vi "Nav_CheckMinDistanceToNode.vi"(9 "Array of path nodes":T1, 11 "Robot current position":T2) -> (3 "Coordinates":T1)   [LabVIEW 2009, in "Navigation.lvlib"]
uses:
  Navigation.lvlib
  Nav_CordinateArray.ctl
  Drive/Drive_Utils.lvlib
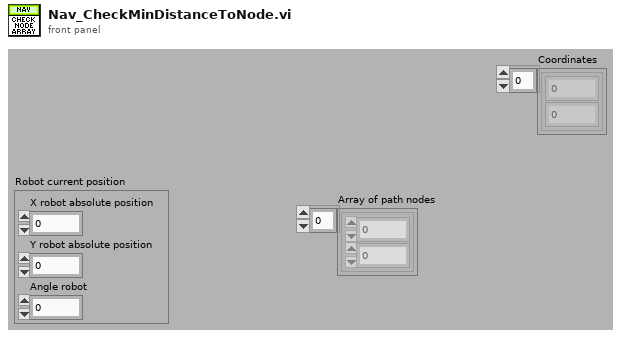
[diagram p1: front panel]
types:
  T1 = typedef "Navigation.lvlib/Nav_CordinateArray.ctl" = cluster{"X position":dbl, "Y position":dbl}[]
  T2 = cluster{"X robot absolute position":dbl, "Y robot absolute position":dbl, "Angle robot":dbl}
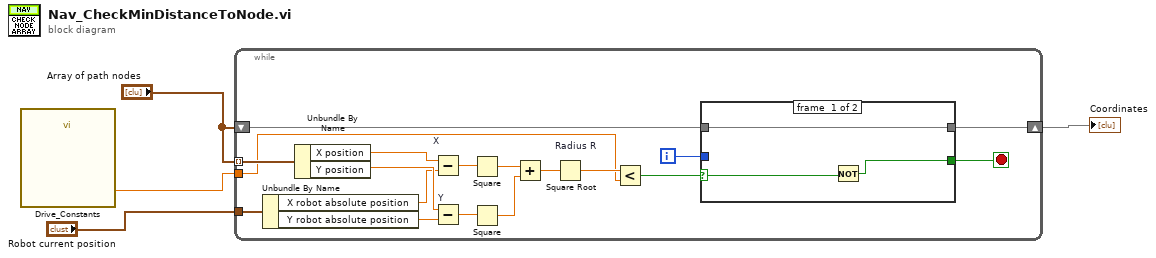
[diagram p0: block diagram]
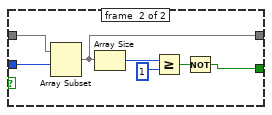
[diagram p2: hidden frame]
diagram:
  n1 = call "Drive_Constants.vi"() -> ("Position accuracy (m)"=w2:dbl)  [unwired: 20 in, 7 out]
  n2 = while {
    tunnel: "Array of path nodes" -> [w21] mode=indexing
    shift-right: [w7] -> w1
    shift-left: "Array of path nodes" -> [w8]
    tunnel: "Robot current position" -> [w22]
    tunnel: w2 -> [w9]
    i -> [w6]
    stop <- w5 stop-if-true
    n3 = Unbundle By Name(w22) -> ("X robot absolute position"=w12:dbl, "Y robot absolute position"=w15:dbl)
    n4 = Unbundle By Name(w21) -> ("X position"=w13:dbl, "Y position"=w14:dbl)
    n5 = Subtract "X"(x=w13, y=w12) -> (x-y=w17:dbl)
    n6 = Subtract "Y"(x=w14, y=w15) -> (x-y=w16:dbl)
    n7 = Square(x=w17) -> (x^2=w20:dbl)
    n8 = Square(x=w16) -> (x^2=w18:dbl)
    n9 = Add(x=w20, y=w18) -> (x+y=w19:dbl)
    n10 = Square Root "Radius R"(x=w19) -> (sqrt(x)=w11:dbl)
    n11 = Less?(x=w11, y=w9) -> (x < y?=w10:bool)
    n12 = case shown="False" w10 {
      selector: w10 -> [w25 _]
      tunnel: w8 -> [w23 w32]
      tunnel: [w23 w28] -> w7
      tunnel: w6 -> [_ w31]
      tunnel: [w24 w26] -> w5
      frame #0 {
        n13 = Not(x=w25) -> (.not. x?=w24:bool)
      }
      frame #1 {
        n14 = Array Subset(array=w32, index=w31) -> (w28:T1)  [unwired: 1 in]
        n15 = Array Size(array=w28) -> (size(s)=w29:i32)
        n16 = Greater Or Equal?(x=w29, y=1) -> (x >= y?=w27:bool)
        n17 = Not(x=w27) -> (.not. x?=w26:bool)
      }
    }
  }
  "Coordinates" <- w1
